vi "Set Handle.vi"(8 "error in (no error)":errorcluster, 10 "handle index":i32, 11 "CCDCamera in":refnum<class "CCDCamera.lvclass">) -> (0 "error out":errorcluster, 3 "CCDCamera out":refnum<class "CCDCamera.lvclass">)   [LabVIEW 2018, in "CCDCamera.lvclass"]
uses:
  CCDCamera.lvclass
  C:/Users/observer/Desktop/SPARC4_ACS/SPARC4_ACS/Simulated_CCD_Camera/Simulated_CCD_Camera.lvclass
  Simulated_CCD_Camera/Simulated_CCD_Camera.lvclass
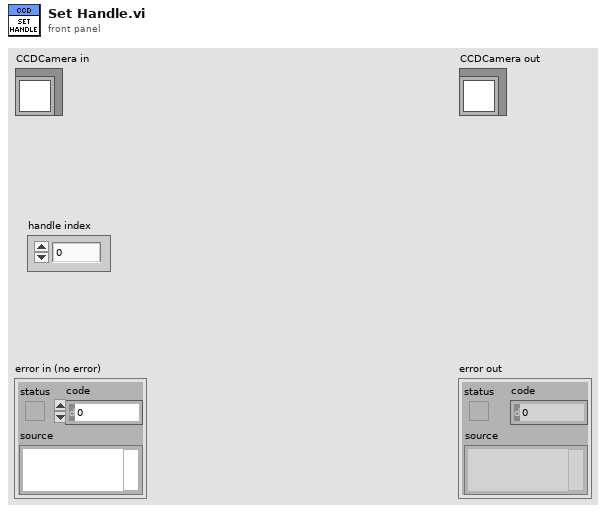
[diagram p1: front panel]
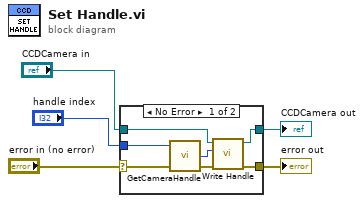
[diagram p0: block diagram]
diagram:
  n1 = case shown="No Error" "error in (no error)" {
    selector: "error in (no error)" -> [w12 w13]
    tunnel: [w8 w13] -> w4
    tunnel: "handle index" -> [w6 _]
    tunnel: "CCDCamera in" -> [w11 w14]
    tunnel: [w7 w14] -> w1
    frame No Error {
      n2 = call <userlib>:"GetCameraHandle.vi"("error in (no error)"=w12, "cameraIndex"=w6) -> ("error out"=w9:errorcluster, "cameraHandle"=w10:i32)  [unwired: 1 in, 1 out]
      n3 = call "Write Handle.vi"("error in (no error)"=w9, "Handle"=w10, "Simulated_CCD_Camera in"=w11) -> ("error out"=w8:errorcluster, "Simulated_CCD_Camera out"=w7:refnum<class "Simulated_CCD_Camera.lvclass">)  [unwired: 7 in]
    }
    frame Error {
    }
  }
  "error out" <- w4
  "CCDCamera out" <- w1
